vi "graph_1d_control.vi"() -> ()   [LabVIEW 2020]
panel:
  out "Y":dbl[](array[numeric])
  in  "graph":dbl[](graph)
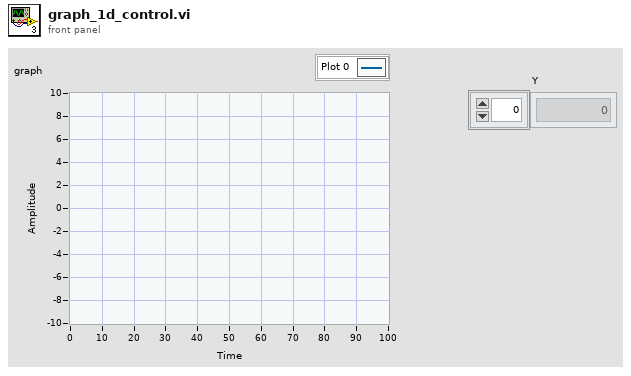
[diagram p1: front panel]
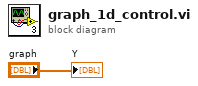
[diagram p0: block diagram]
diagram:
  "Y" <- "graph"
